vi "Escape YAML.vi"(8 "error in (no error)":errorcluster, 11 "String":string) -> (0 "error out":errorcluster, 3 "YAML String":string)   [LabVIEW 2015, in "YAML Parser.lvclass"]
uses:
  YAML Parser.lvclass
panel:
  in  "Level":u32
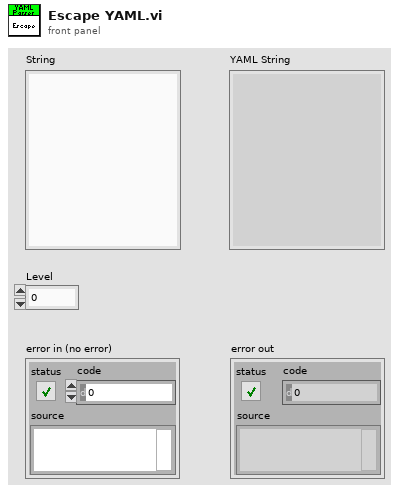
[diagram p1: front panel]
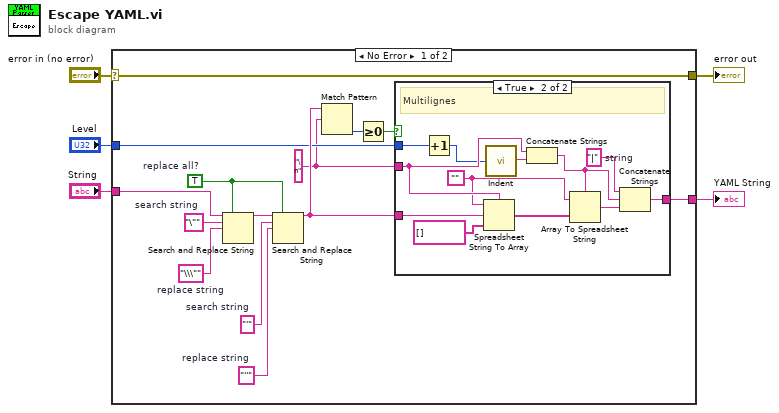
[diagram p0: block diagram]
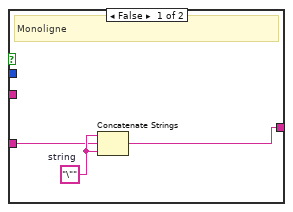
[diagram p2: hidden frame]
diagram:
  n1 = case shown="No Error" "error in (no error)" {
    selector: "error in (no error)" -> [w19 w35]
    tunnel: [w19 w35] -> w4
    tunnel: "String" -> [w18 w36]
    tunnel: [w9 w36] -> w2
    tunnel: "Level" -> [w7 _]
    frame No Error {
      w6 = "\n"
      w13 = "'"  # search string
      w12 = "''"  # replace string
      w14 = TRUE  # replace all?
      w16 = "\\\""  # replace string
      w17 = "\""  # search string
      n2 = Search and Replace String(replace all?=w14, input string=w18, search string=w17, replace string=w16) -> (result string=w15:string)  [unwired: 4 in, 3 out]
      n3 = Search and Replace String(replace all?=w14, input string=w15, search string=w13, replace string=w12) -> (result string=w8:string)  [unwired: 4 in, 3 out]
      n4 = Match Pattern(string=w8, regular expression=w6) -> (offset past match=w11:i32)  [unwired: 1 in, 3 out]
      n5 = Greater Or Equal To 0?(x=w11) -> (x >= 0?=w10:bool)
      n6 = case shown="True" w10 {
        tunnel: [w20 w31] -> w9
        tunnel: w8 -> [w21 w25]
        tunnel: w7 -> [_ w32]
        tunnel: w6 -> [_ w27]
        frame False {
          w22 = "\""  # string
          # "Monoligne"
          n7 = Concatenate Strings(w22, w21, w22) -> (w20:string)
        }
        frame True {
          w26 = ""
          w34 = "|"  # string
          # "Multilignes"
          n8 = Increment(x=w32) -> (x+1=w23:u32)
          n9 = Spreadsheet String To Array(delimiter (Tab)=w27, format string=w26, spreadsheet string=w25, array type (2D Dbl)=string[] []) -> (array=w30:string[])
          n10 = call "Indent.vi"("Index"=w23) -> ("Indentation"=w24:string)
          n11 = Concatenate Strings(w27, w24) -> (w29:string)
          n12 = Array To Spreadsheet String(delimiter (Tab)=w29, array=w30, 3:w26) -> (spreadsheet string=w28:string)
          n13 = Concatenate Strings(w34, w29, w28) -> (w31:string)
        }
      }
    }
    frame Error {
    }
  }
  "error out" <- w4
  "YAML String" <- w2
